vi "Prober_ValidCoordinate.vi"(8 "error in (no error)":errorcluster, 9 "Axis":enum16{"X", "Y", "Z", "Theta"}(ring), 10 "Coordinate IN":i32, 11 "AlessiRel6100 in":refnum<class "AlessiRel6100.lvclass">) -> (0 "error out":errorcluster, 2 "Is Valid?":bool, 3 "AlessiRel6100 out":refnum<class "AlessiRel6100.lvclass">)   [LabVIEW 2018, in "AlessiRel6100.lvclass"]
uses:
  AlessiRel6100.lvclass
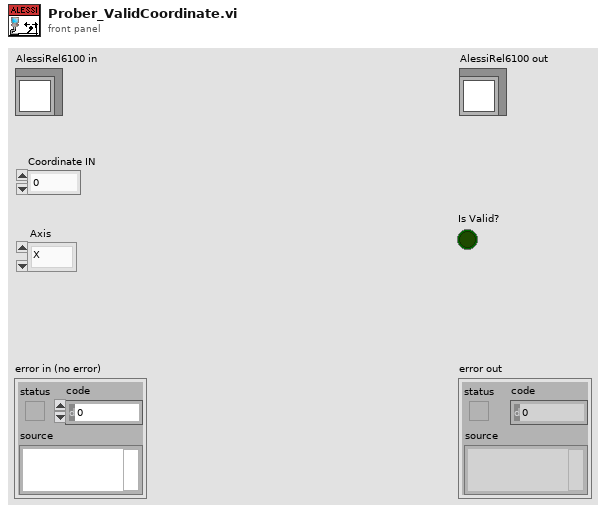
[diagram p1: front panel]
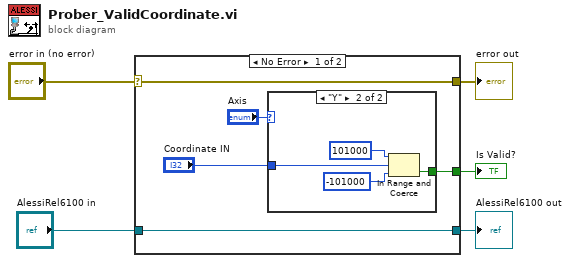
[diagram p0: block diagram]
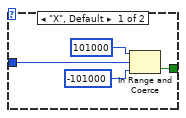
[diagram p2: hidden frame]
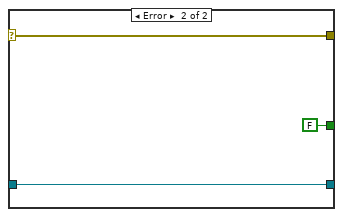
[diagram p3: hidden frame]
diagram:
  n1 = case shown="No Error" "error in (no error)" {
    selector: "error in (no error)" -> [w10 w20]
    tunnel: [w10 w20] -> w4
    tunnel: "AlessiRel6100 in" -> [w9 w21]
    tunnel: [w9 w21] -> w2
    tunnel: [w8 FALSE] -> w1
    frame No Error {
      n2 = case shown="\"Y\"" "Axis" {
        tunnel: [w11 w16] -> w8
        tunnel: "Coordinate IN" -> [w13 w15]
        frame "X", Default {
          n3 = In Range and Coerce(upper limit=101000, x=w13, lower limit=-101000) -> (In Range?=w11:bool)  [unwired: 1 out]
        }
        frame "Y" {
          n4 = In Range and Coerce(upper limit=101000, x=w15, lower limit=-101000) -> (In Range?=w16:bool)  [unwired: 1 out]
        }
      }
    }
    frame Error {
    }
  }
  "error out" <- w4
  "AlessiRel6100 out" <- w2
  "Is Valid?" <- w1
